vi "Handle Error.vi"(8 "error in (no error)":errorcluster, 11 "Elevator Controller in":refnum<class "Elevator Controller.lvclass">) -> (0 "error out":errorcluster, 2 "stop actor?":bool=TRUE, 3 "Elevator Controller out":refnum<class "Elevator Controller.lvclass">)   [LabVIEW 2019, in "Elevator Controller Actor.lvlib" / "Elevator Controller.lvclass"]
doc: "(<B>Filename</B>: Actor Framework.lvlib:Actor.lvclass:Handle Error.vi)\n\nDefines how the actor handles an error that occurred while processing a message. By default, this method does nothing except stop the actor."
uses:
  Elevator Controller.lvclass
  <vilib>/ActorFramework/Actor/Actor.lvclass
  Elevator Controller Messages/Set State Msg/Set State Msg.lvclass
  States -Enum.ctl
  C:/Program Files (x86)/National Instruments/LabVIEW 2019/vi.lib/ActorFramework/Actor/Actor.lvclass
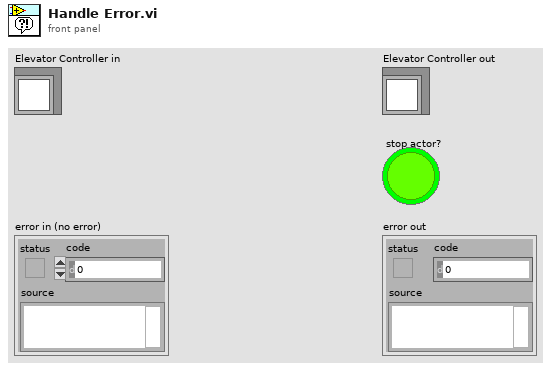
[diagram p1: front panel]
types:
  T1 = typedef "Elevator Controller Actor.lvlib/Elevator Controller.lvclass/States -Enum.ctl" = enum16{"Initial State", "Start and Move State", "Analysis State", "Continue Travel State", "Open and Close Door Sequence", "Stop at Floor", "No Request remaining", "Emergency Call", "Terminate Process"}
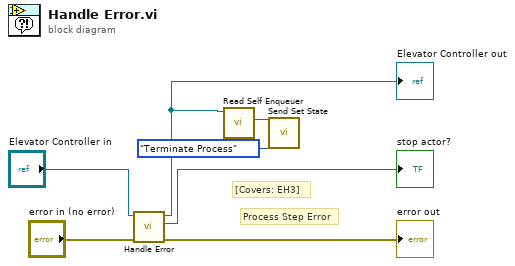
[diagram p0: block diagram]
diagram:
  # "Process Step Error"
  # "[Covers: EH3]"
  n1 = call-parent "Handle Error.vi"("error in (no error)"="error in (no error)", "Actor in"="Elevator Controller in") -> ("error out"=→"error out":errorcluster, "stop actor?"=→"stop actor?":bool, "Actor out"=w3:refnum<class "Elevator Controller.lvclass">)  [unwired: 7 in]
  "Elevator Controller out" <- w3
  n2 = call <vilib>:"Read Self Enqueuer.vi"("Actor"=w3) -> ("Self Enqueuer"=w2:refnum<class "Message Enqueuer.lvclass">)  [unwired: 10 in]
  n3 = call "Send Set State.vi"("States"=States_-Enum."Terminate Process", "Message Enqueuer"=w2) -> ()  [unwired: 8 in, 2 out]
